vi "Calculate Sidebar Centered Text x.vi"(9 "Width":i32, 10 "Sidebar Width":i32, 11 "x":i32) -> (3 "Numeric":i32)   [LabVIEW 2021, in "Ship.lvclass"]
uses:
  Ship.lvclass
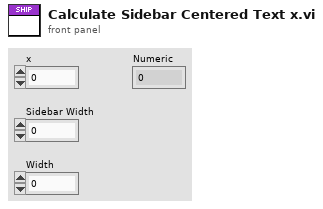
[diagram p1: front panel]
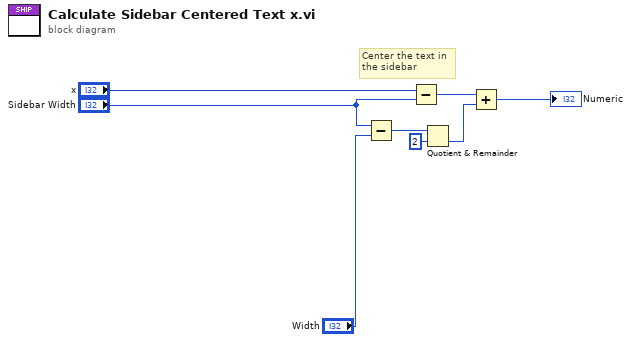
[diagram p0: block diagram]
diagram:
  # "Center the text in the sidebar"
  n1 = Subtract(x="Sidebar Width", y="Width") -> (x-y=w5:i32)
  n2 = Subtract(x="x", y="Sidebar Width") -> (x-y=w2:i32)
  n3 = Quotient & Remainder(x=w5, y=2) -> (floor(x/y)=w7:i32)  [unwired: 1 out]
  n4 = Add(x=w2, y=w7) -> (x+y=→"Numeric":i32)
